vi "Actor Core.vi"(8 "error in":errorcluster, 11 "Child_1 in":refnum<class "SW_Interface_Class.lvclass">) -> (0 "error out":errorcluster, 3 "Actor out":refnum<class "Actor.lvclass">)   [LabVIEW 2023, in "SW_Interface_Actor.lvlib" / "SW_Interface_Class.lvclass"]
doc: "(<B>Filename</B>: Actor Framework.lvlib:Actor.lvclass:Actor Core.vi)\n\nReceives messages to the actor, reacts to them, and initiates any error handling that may shut the actor down.\n\nDescendant classes may override this VI to append parallel tasks for the actor to complete while it handles messages. Overrides use the Call Parent Class Method node."
uses:
  SW_Interface_Class.lvclass
  <vilib>/ActorFramework/Actor/Actor.lvclass
  SW_Interface_Class.lvclass/SW_Interface_Class.ctl
  Abstraction_Interface_Class/Abstraction_Interface_Class.lvclass
panel:
  out "RAW_Actor_Name":string
  in  "Console":string
  # "SW INTERFACE"
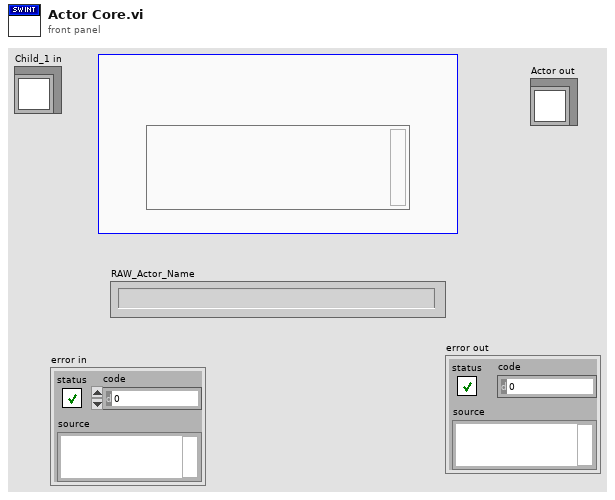
[diagram p1: front panel]
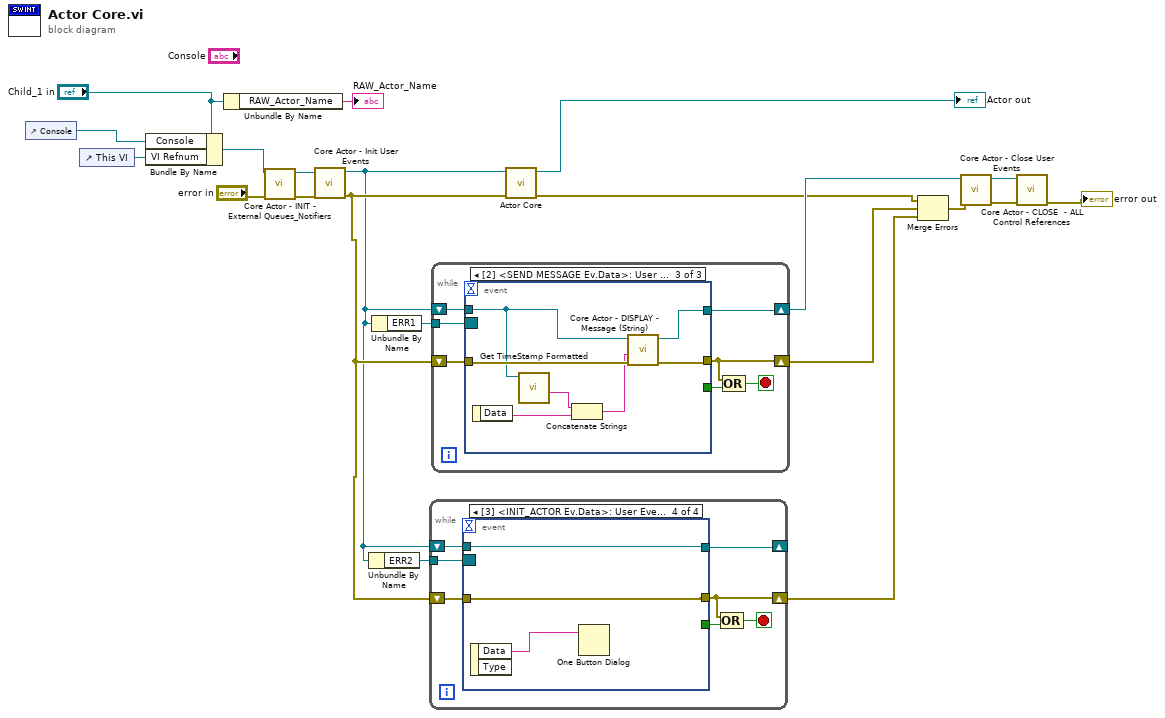
[diagram p0: block diagram]
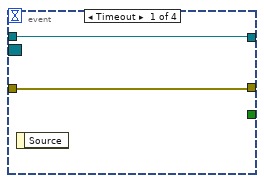
[diagram p2: hidden frame]
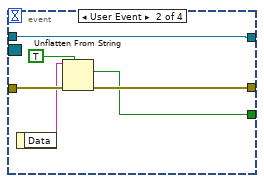
[diagram p3: hidden frame]
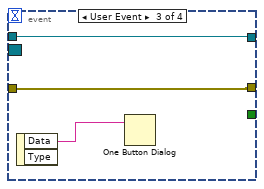
[diagram p4: hidden frame]
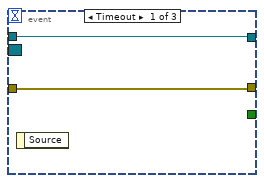
[diagram p5: hidden frame]
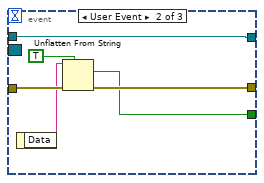
[diagram p6: hidden frame]
diagram:
  n1 = control-ref of="Console"() -> (w8:refnum<vi>)
  n2 = control-ref of="This VI"() -> (w9:refnum<vi>)
  n3 = Bundle By Name(cluster="Child_1 in", "Console"=w8, "VI Refnum"=w9) -> (w7:refnum<class "SW_Interface_Class.lvclass">)
  n4 = Unbundle By Name("Child_1 in") -> ("RAW_Actor_Name"=→"RAW_Actor_Name":string)
  n5 = call-dynamic "Core Actor - INIT - External Queues_Notifiers.vi"("error in (no error)"="error in", "Child_2_Class in"=w7) -> ("error out"=w19:errorcluster, "Child_2_Class out"=w18:refnum<class "SW_Interface_Class.lvclass">)  [unwired: 8 in]
  n6 = call-dynamic "Core Actor - Init User Events.vi"("error in (no error)"=w19, "Child_2_Class in"=w18) -> ("error out"=w5:errorcluster, "Child_2_Class out"=w4:refnum<class "SW_Interface_Class.lvclass">)  [unwired: 8 in]
  n7 = Unbundle By Name(w4) -> ("ERR2"=w6:refnum<event-registration>)
  n8 = Unbundle By Name(w4) -> ("ERR1"=w14:refnum<event-registration>)
  n9 = while {
    shift-right: [w24] -> w3
    shift-left: w5 -> [w26]
    shift-right: [w27] -> _
    shift-left: w4 -> [w28]
    tunnel: w6 -> [w25]
    stop <- w22 stop-if-true
    n10 = event shown="[3] <INIT_ACTOR Ev.Data>: User Event" {
      selector: w25 -> [_ _ _ _]
      dyn-events: _ -> [_ _ _ _]
      timeout: _ -> [_ _ _ _]
      tunnel: w28 -> [w30 w31 w39 w42]
      tunnel: [w30 w31 w39 w42] -> w27
      tunnel: w26 -> [w29 w36 w38 w41]
      tunnel: [w29 w33 w38 w41] -> w24
      tunnel: [_ w32 _ _] -> w23
      event Timeout {
        n11 = event-data() -> ()  [unwired: 1 in, 1 out]
      }
      event User Event {
        n12 = event-data() -> ("Data"=w35:string)  [unwired: 1 in]
        n13 = Unflatten From String(type=TRUE, binary string=w35, error in (no error)=w36) -> (value=w32:bool, error out=w33:errorcluster)  [unwired: 2 in, 1 out]
      }
      event User Event {
        n14 = event-data() -> ("Data"=w37:string)  [unwired: 1 in, 1 out]
        n15 = One Button Dialog(message=w37) -> ()  [unwired: 1 in, 1 out]
      }
      event User Event {
        n16 = event-data() -> ("Data"=w40:string)  [unwired: 1 in, 1 out]
        n17 = One Button Dialog(message=w40) -> ()  [unwired: 1 in, 1 out]
      }
    }
    n18 = Compound Arithmetic op=OR(w24, w23) -> (w22:bool)
  }
  n19 = while {
    shift-right: [w45] -> w13
    shift-left: w5 -> [w47]
    shift-right: [w48] -> w12
    shift-left: w4 -> [w49]
    tunnel: w14 -> [w46]
    stop <- w43 stop-if-true
    n20 = event shown="[2] <SEND MESSAGE Ev.Data>: User Event" {
      selector: w46 -> [_ _ _]
      dyn-events: _ -> [_ _ _]
      timeout: _ -> [_ _ _]
      tunnel: w49 -> [w51 w52 w61]
      tunnel: [w51 w52 w62] -> w48
      tunnel: w47 -> [w50 w57 w64]
      tunnel: [w50 w54 w63] -> w45
      tunnel: [_ w53 _] -> w44
      event Timeout {
        n21 = event-data() -> ()  [unwired: 1 in, 1 out]
      }
      event User Event {
        n22 = event-data() -> ("Data"=w56:string)  [unwired: 1 in]
        n23 = Unflatten From String(type=TRUE, binary string=w56, error in (no error)=w57) -> (value=w53:bool, error out=w54:errorcluster)  [unwired: 2 in, 1 out]
      }
      event User Event {
        n24 = event-data() -> ("Data"=w59:string)  [unwired: 1 in]
        n25 = call-dynamic "Get TimeStamp Formatted.vi"("Child_2_Class in"=w61) -> ("TimeStamp Formatted"=w60:string)  [unwired: 8 in, 2 out]
        n26 = Concatenate Strings(w60, w59) -> (w58:string)
        n27 = call-dynamic "Core Actor - DISPLAY - Message (String).vi"("error in (no error)"=w64, "Value"=w58, "Interface_Class in"=w61) -> ("error out"=w63:errorcluster, "Interface_Class out"=w62:refnum<class "SW_Interface_Class.lvclass">)  [unwired: 7 in]
      }
    }
    n28 = Compound Arithmetic op=OR(w45, w44) -> (w43:bool)
  }
  n29 = call-parent "Actor Core.vi"("error in"=w5, "Actor in"=w4) -> ("error out"=w10:errorcluster, "Actor out"=→"Actor out":refnum<class "Actor.lvclass">)  [unwired: 8 in]
  n30 = Merge Errors(w10, w13, w3) -> (w11:errorcluster)
  n31 = call-dynamic "Core Actor - Close User Events.vi"("error in (no error)"=w11, "Interface_Class in"=w12) -> ("error out"=w17:errorcluster, "Interface_Class out"=w16:refnum<class "SW_Interface_Class.lvclass">)  [unwired: 8 in]
  n32 = call-dynamic "Core Actor - CLOSE  - ALL Control References.vi"("error in (no error)"=w17, "Child_2_Class in"=w16) -> ("error out"=→"error out":errorcluster)  [unwired: 8 in, 1 out]
